vi "Autonomous Independent.vi"() -> ()   [LabVIEW 2013]
doc: "This VI is called when autonomous begins, and will automatically be terminated when autonomous ends. You can carry out timed or sensor driven robot movement independently without needing to return to the caller."
uses:
  Autonomous State.ctl
  <vilib>/Rock Robotics/WPI/Solenoid/WPI_SolenoidValue.ctl
  <vilib>/Rock Robotics/WPI/DriverStation/WPI_DriverStationRobotMode2.ctl
  Robot Global Data.vi
  <vilib>/Rock Robotics/WPI/Solenoid/WPI_SolenoidSetEnum.vi
  <vilib>/Rock Robotics/WPI/RobotDrive/WPI_RobotDriveGetSetRefNum.vi
  <vilib>/Rock Robotics/WPI/RobotDrive/WPI_RobotDriveArcadeDrive_Standard(NoSaturation).vi
panel:
  out "Enum":T1
  # "Be sure to right-click and choose Data Operations>>Make Current Value default if you want to save the array values with the VI"
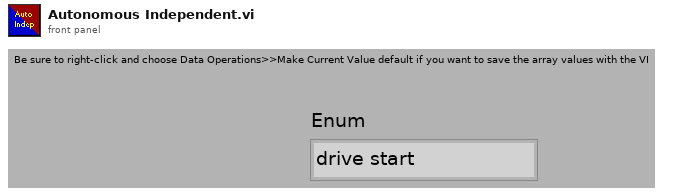
[diagram p1: front panel]
types:
  T1 = typedef "Autonomous State.ctl" = enum16{"drive start", "drive stop", "One Ball: Shoot", "reload", "One Ball: Look for target", "retract arm", "drive faster", "drive time for 2ball", "turn", "One Ball: Finish", "Two Ball: First shoot", "Two Ball: Grab second ball", "Two Ball: Second shoot", "Two Ball: Finish"}
  T2 = typedef "WPI_SolenoidDevRef.ctl" = cluster{"DevStatus":errorcluster, "Solenoid Module":T3, "Forward Solenoid Channel":T4, "Reverse Solenoid Channel":T4}
  T3 = typedef "FPGA_TypedefSolenoidModule.ctl" = enum16{"Solenoid Module 1", "Solenoid Module 2"}
  T4 = typedef "WPI_SolenoidChannel.ctl" = enum8{"Solenoid 1", "Solenoid 2", "Solenoid 3", "Solenoid 4", "Solenoid 5", "Solenoid 6", "Solenoid 7", "Solenoid 8", "Invalid"}
  T5 = typedef "WPI_DriverStationRobotMode2.ctl" = enum16{"Autonomous Disabled", "Autonomous Enabled", "Teleop Disabled", "Teleop Enabled", "Timeout", "Finish", "Test Disabled", "Test Enabled"}
  T6 = typedef "WPI_SolenoidValue.ctl" = enum16{"Off", "On", "Forward", "Reverse"}
  T7 = typedef "WPI_MotorControlDeviceRef.ctl" = cluster{"DeviceStatus":errorcluster, "Type":enum16{"PWM", "CAN"}, "PWM":cluster{"Digital Module":T8, "PWM Channel":T9, "DeadBand":T10}, "CAN":cluster{"Device Number":u8, "Control Mode":T11, "Semaphore":T12, "Max Vout":dbl}, "Invert":bool, "TransformRef":T13, "InvTransformRef":T13}
  T8 = typedef "FPGA_TypedefDigitalModule.ctl" = enum16{"Digital Module 1", "Digital Module 2"}
  T9 = typedef "FPGA_DIOPWMChannel.ctl" = enum8{"PWM 1", "PWM 2", "PWM 3", "PWM 4", "PWM 5", "PWM 6", "PWM 7", "PWM 8", "PWM 9", "PWM 10", "Invalid"}
  T10 = typedef "WPI_PWMDeadband.ctl" = cluster{"Name":string, "maxPositivePwm":i32, "minPositivePwm":i32, "centerPwm":i32, "maxNegativePwm":i32, "minNegativePwm":i32, "angularRange":u16}
  T11 = typedef "WPI_CANJaguar_ControlMode.ctl" = enum8{"Percent VBus", "Current", "Speed", "Position", "Voltage"}
  T12 = typedef "Semaphore RefNum" = refnum<k1>
  T13 = typedef "WPI_PWMTransform_ConPane.ctl" = refnum<vi>
  T14 = typedef "WPI_DigitalInputDevRef.ctl" = cluster{"DevStatus":errorcluster, "DIO Channel":T15, "Digital Module":T8}
  T15 = typedef "FPGA_DIOChannel.ctl" = enum8{"DIO 1", "DIO 2", "DIO 3", "DIO 4", "DIO 5", "DIO 6", "DIO 7", "DIO 8", "DIO 9", "DIO 10", "DIO 11", "DIO 12", "DIO 13", "DIO 14", "Invalid"}
  T16 = typedef "WPI_RobotDriveDevRef.ctl" = cluster{"DevStatus":errorcluster, "Motors[]":T7[], "Square Inputs":bool, "Max Output":dbl, "Isochronous":bool}
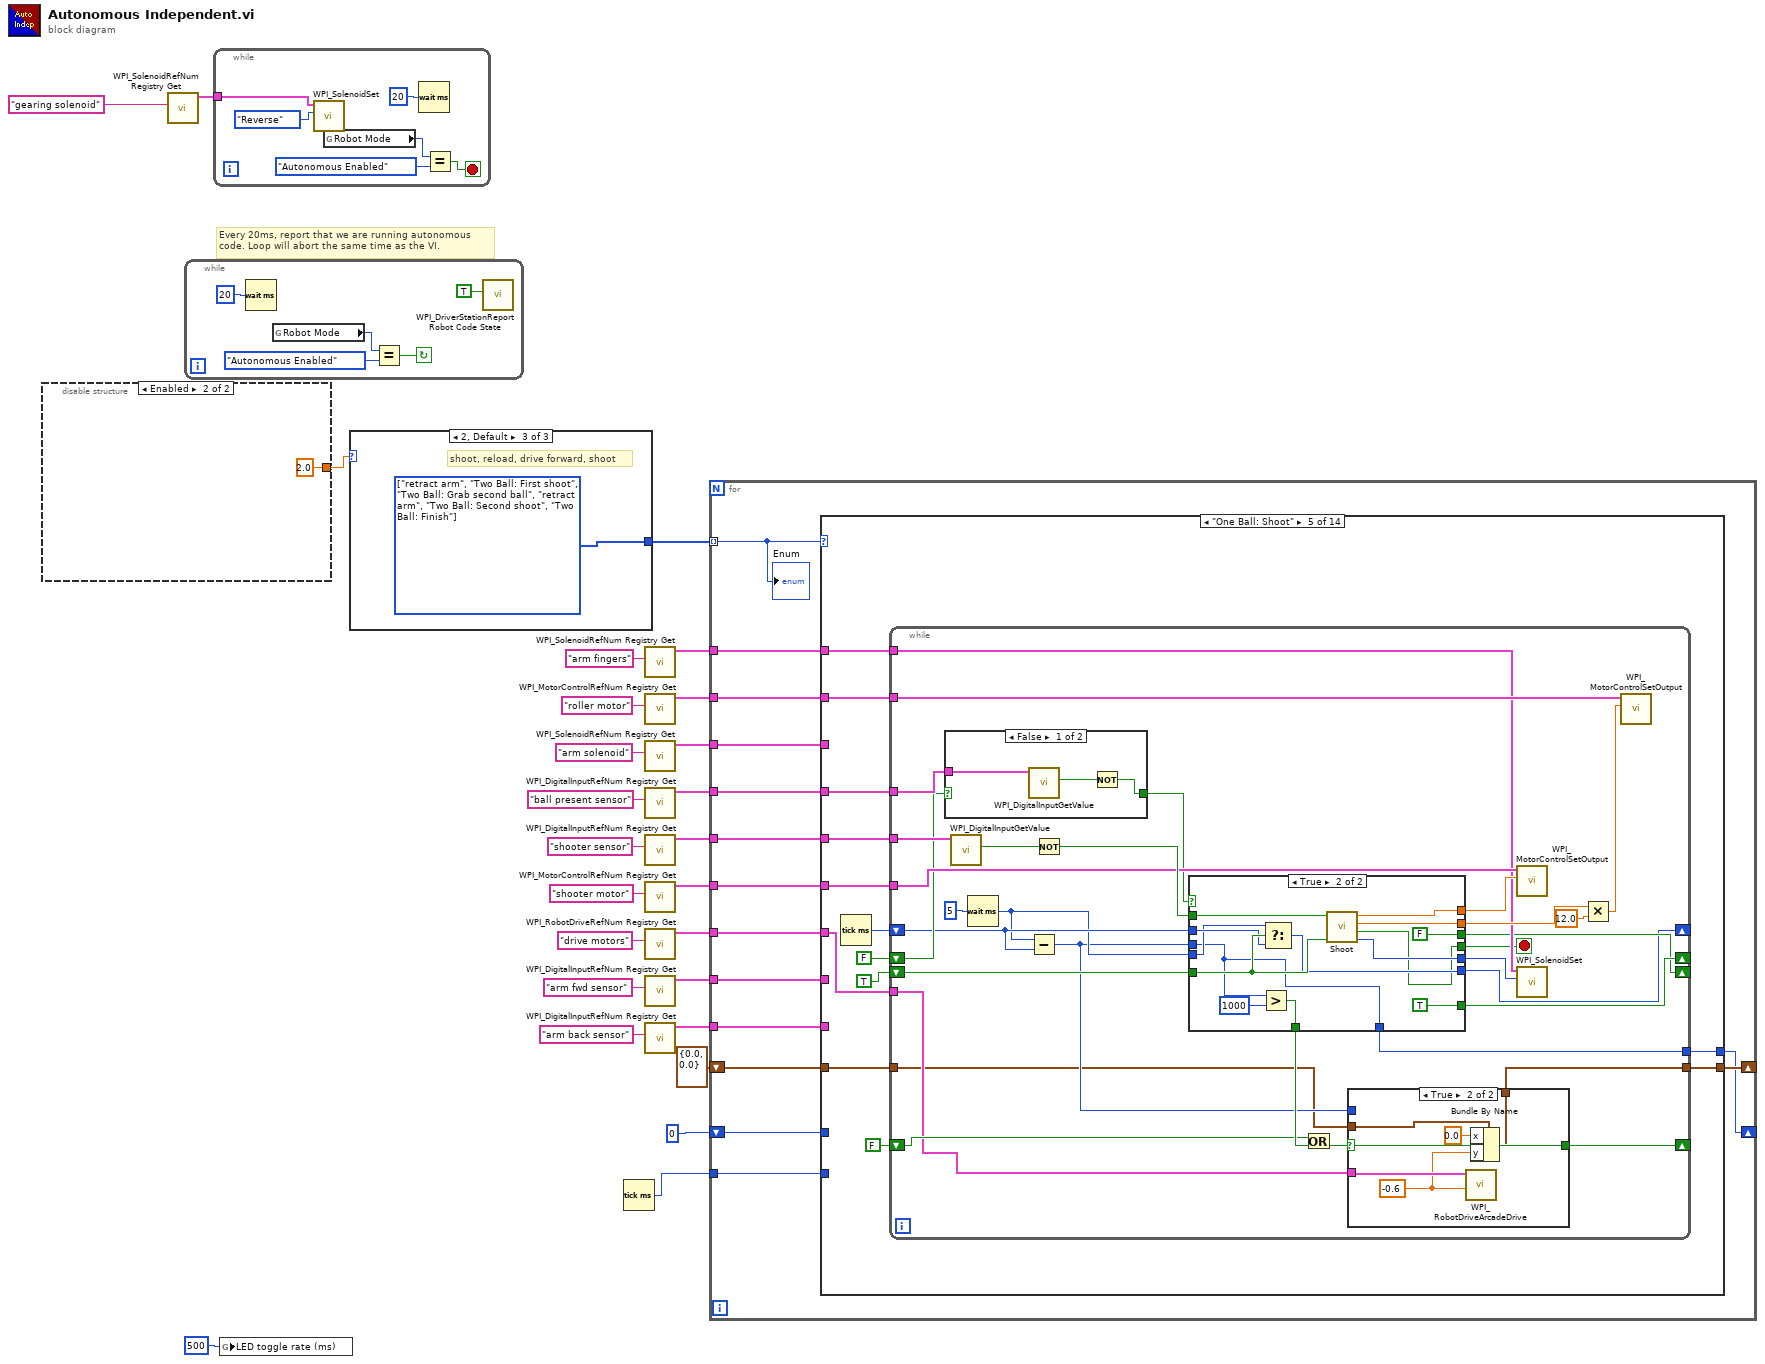
[diagram p0: block diagram]
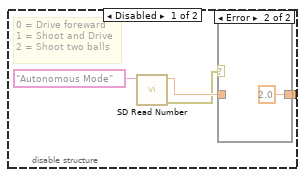
[diagram p2: hidden frame]
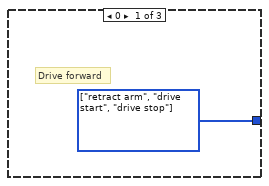
[diagram p4: hidden frame]
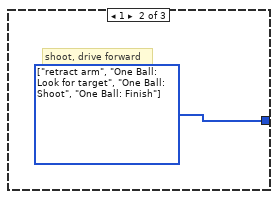
[diagram p5: hidden frame]
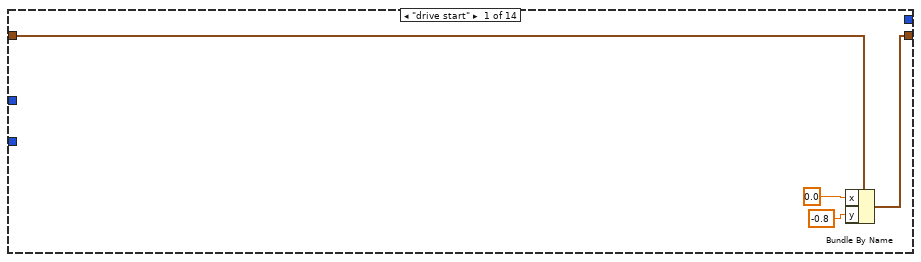
[diagram p6: hidden frame]
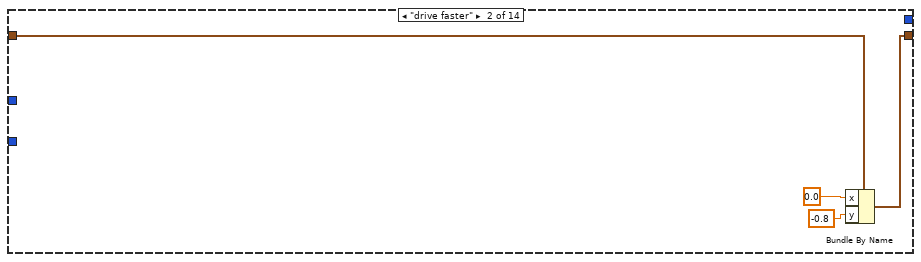
[diagram p7: hidden frame]
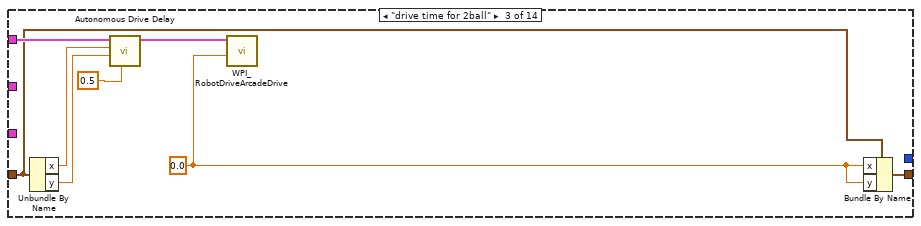
[diagram p8: hidden frame]
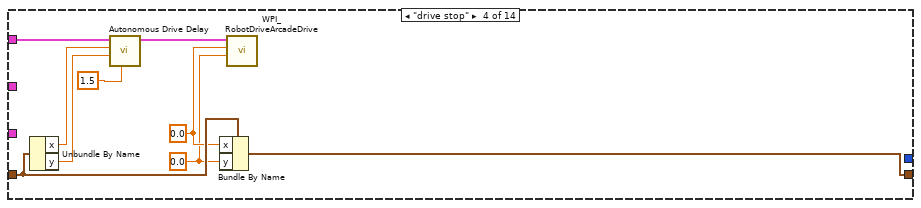
[diagram p9: hidden frame]
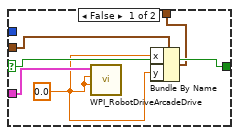
[diagram p10: hidden frame]
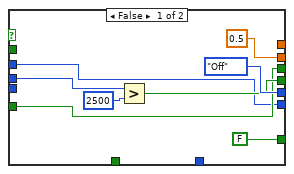
[diagram p12: hidden frame]
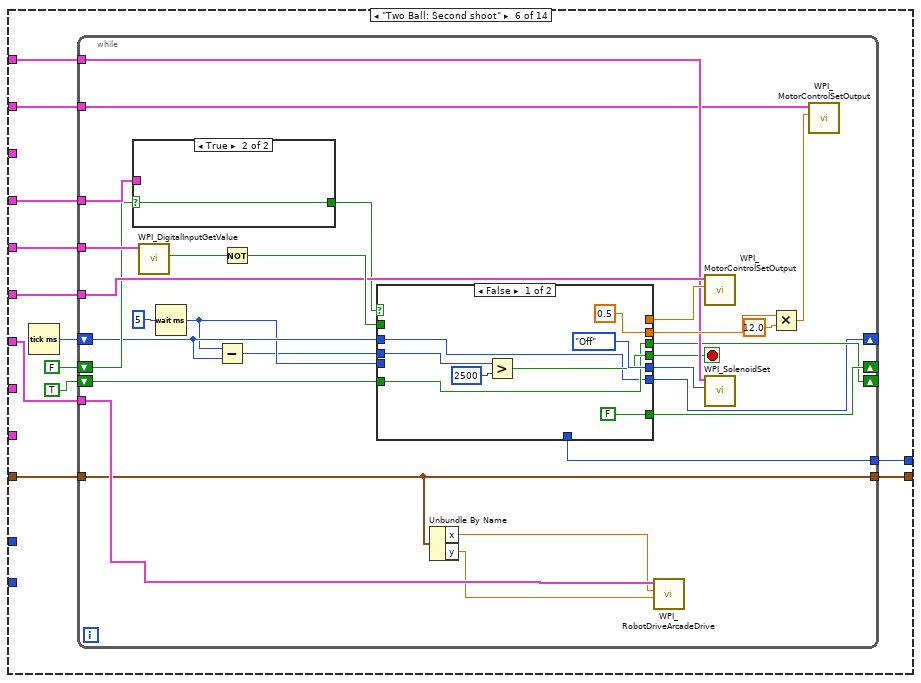
[diagram p13: hidden frame]
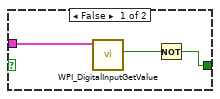
[diagram p14: hidden frame]
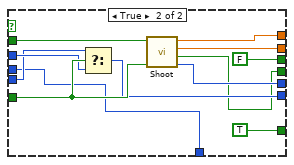
[diagram p15: hidden frame]
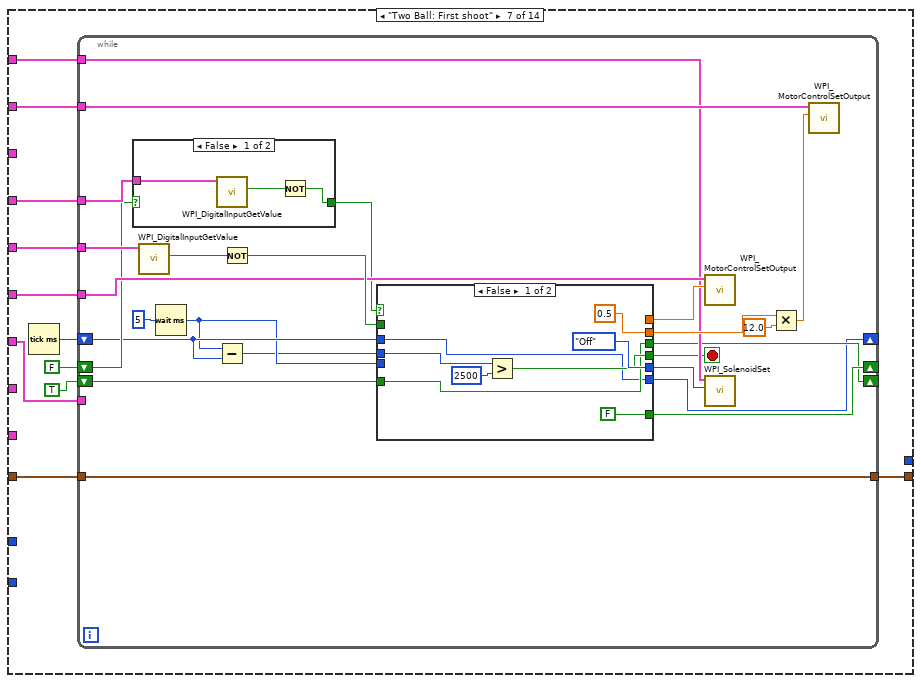
[diagram p16: hidden frame]
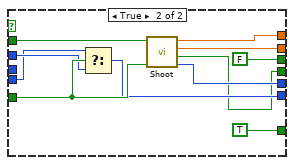
[diagram p18: hidden frame]
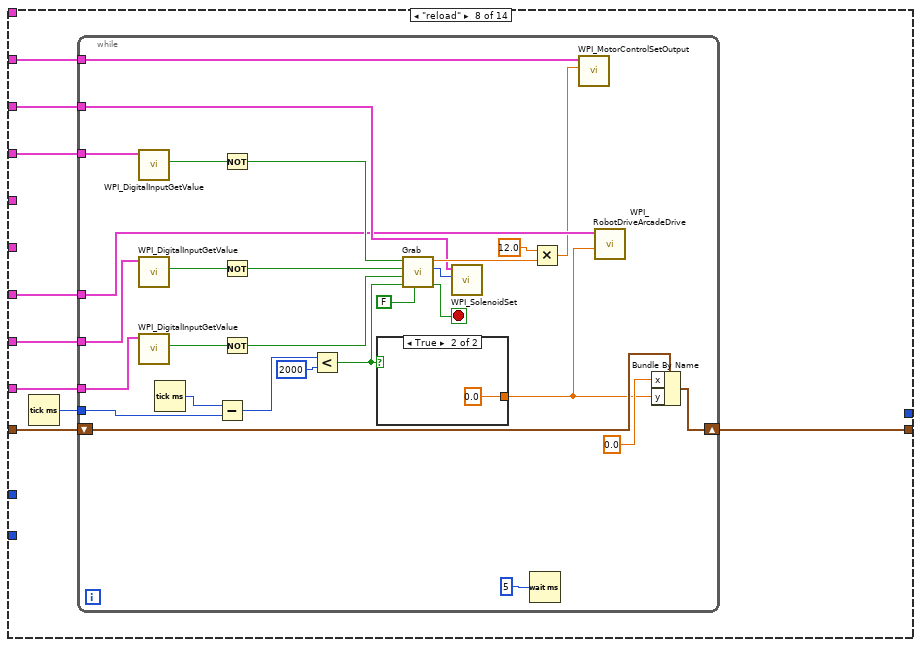
[diagram p19: hidden frame]
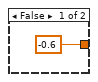
[diagram p20: hidden frame]
diagram:
  # "Every 20ms, report that we are running autonomous\ncode. Loop will abort the same time as the VI."
  n1 = disable-structure shown="Enabled" {
    disable-tunnel: [w29 2.0 ("Numeric")] -> w1
    frame Disabled {
      # "0 = Drive foreward\n1 = Shoot and Drive\n2 = Shoot two balls"
      n2 = call <vilib>:"SD Read Number.vi"("Name"="Autonomous Mode") -> ("error out"=w27:errorcluster, "Numeric"=w28:dbl)  [unwired: 8 in, 1 out]
      n3 = case shown="Error" w27 {
        tunnel: [w31 2.0 ("Numeric")] -> w29
        tunnel: w28 -> [w31 _]
        frame No Error {
        }
        frame Error {
        }
      }
    }
    frame Enabled {
    }
  }
  n4 = call <vilib>:"WPI_SolenoidRefNum Registry Get.vi"("refnum name"="gearing solenoid") -> ("SolenoidDevRef"=w2:T2)  [unwired: 9 in, 1 out]
  n5 = while {
    stop <- w34 continue-if-true
    n6 = Wait (ms)(milliseconds to wait=u32 20) -> ()  [unwired: 1 out]
    n7 = global read "Robot Global Data.vi" "Robot Mode"() -> (w36:T5)
    n8 = Equal?(x=w36, y=WPI_DriverStationRobotMode2."Autonomous Enabled") -> (x = y?=w34:bool)
    n9 = call <vilib>:"WPI_DriverStationReport Robot Code State.vi"("Autonomous"=TRUE) -> ()  [unwired: 10 in, 1 out]
  }
  n10 = while {
    tunnel: w2 -> [w43]
    stop <- w40 stop-if-true
    n11 = call-poly <vilib>:"WPI_SolenoidSet.vi"("Value"=WPI_SolenoidValue."Reverse", "SolenoidDevRef"=w43) -> ()  [unwired: 8 in, 2 out]
    n12 = global read "Robot Global Data.vi" "Robot Mode"() -> (w41:T5)
    n13 = Wait (ms)(milliseconds to wait=u32 20) -> ()  [unwired: 1 out]
    n14 = Equal?(x=w41, y=WPI_DriverStationRobotMode2."Autonomous Enabled") -> (x = y?=w40:bool)
  }
  n15 = global write "Robot Global Data.vi" "LED toggle rate (ms)"(u32 500 ("LED ms toggle rate")) -> ()
  n16 = case shown="2, Default" w1 {
    tunnel: [w45 w46 w47] -> w7
    frame 0 {
      w45 = T1[] [enum."retract arm", enum."drive start", enum."drive stop"] items=["drive start", "drive stop", "One Ball: Shoot", "reload", "One Ball: Look for target", "retract arm", "drive faster", "drive time for 2ball", "turn", "One Ball: Finish", "Two Ball: First shoot", "Two Ball: Grab second ball", "Two Ball: Second shoot", "Two Ball: Finish"]
      # "Drive forward"
    }
    frame 1 {
      w46 = T1[] [enum."retract arm", enum."One Ball: Look for target", enum."One Ball: Shoot", enum."One Ball: Finish"] items=["drive start", "drive stop", "One Ball: Shoot", "reload", "One Ball: Look for target", "retract arm", "drive faster", "drive time for 2ball", "turn", "One Ball: Finish", "Two Ball: First shoot", "Two Ball: Grab second ball", "Two Ball: Second shoot", "Two Ball: Finish"]
      # "shoot, drive forward"
    }
    frame 2, Default {
      w47 = T1[] [enum."retract arm", enum."Two Ball: First shoot", enum."Two Ball: Grab second ball", enum."retract arm", enum."Two Ball: Second shoot", enum."Two Ball: Finish"] items=["drive start", "drive stop", "One Ball: Shoot", "reload", "One Ball: Look for target", "retract arm", "drive faster", "drive time for 2ball", "turn", "One Ball: Finish", "Two Ball: First shoot", "Two Ball: Grab second ball", "Two Ball: Second shoot", "Two Ball: Finish"]
      # "shoot, reload, drive forward, shoot"
    }
  }
  n17 = Tick Count (ms)() -> (millisecond timer value=w4:u32)
  n18 = call <vilib>:"WPI_SolenoidRefNum Registry Get.vi"("refnum name"="arm fingers") -> ("SolenoidDevRef"=w9:T2)  [unwired: 9 in, 1 out]
  n19 = call <vilib>:"WPI_MotorControlRefNum Registry Get.vi"("refnum name"="roller motor") -> ("MotorControlDevRef"=w14:T7)  [unwired: 9 in, 1 out]
  n20 = call <vilib>:"WPI_SolenoidRefNum Registry Get.vi"("refnum name"="arm solenoid") -> ("SolenoidDevRef"=w13:T2)  [unwired: 9 in, 1 out]
  n21 = call <vilib>:"WPI_DigitalInputRefNum Registry Get.vi"("refnum name"="ball present sensor") -> ("DigitalInputDevRef"=w10:T14)  [unwired: 9 in, 1 out]
  n22 = call <vilib>:"WPI_DigitalInputRefNum Registry Get.vi"("refnum name"="shooter sensor") -> ("DigitalInputDevRef"=w16:T14)  [unwired: 9 in, 1 out]
  n23 = call <vilib>:"WPI_MotorControlRefNum Registry Get.vi"("refnum name"="shooter motor") -> ("MotorControlDevRef"=w15:T7)  [unwired: 9 in, 1 out]
  n24 = call <vilib>:"WPI_RobotDriveRefNum Registry Get.vi"("refnum name"="drive motors") -> ("RobotDriveDevRef"=w17:T16)  [unwired: 9 in, 1 out]
  n25 = call <vilib>:"WPI_DigitalInputRefNum Registry Get.vi"("refnum name"="arm fwd sensor") -> ("DigitalInputDevRef"=w11:T14)  [unwired: 9 in, 1 out]
  n26 = call <vilib>:"WPI_DigitalInputRefNum Registry Get.vi"("refnum name"="arm back sensor") -> ("DigitalInputDevRef"=w12:T14)  [unwired: 9 in, 1 out]
  n27 = for {
    tunnel: w7 -> [w62] mode=indexing
    tunnel: w17 -> [w54]
    tunnel: w16 -> [w61]
    tunnel: w15 -> [w60]
    tunnel: w14 -> [w59]
    tunnel: w13 -> [w58]
    tunnel: w12 -> [w57]
    tunnel: w11 -> [w56]
    tunnel: w10 -> [w55]
    tunnel: w9 -> [w53]
    shift-right: [w51] -> _
    shift-left: cluster{"x":dbl, "y":dbl} {"x"=0.0, "y"=0.0} -> [w52]
    shift-right: [w50] -> _
    shift-left: u32 0 -> [w49]
    tunnel: w4 -> [w48]
    n28 = case shown="\"One Ball: Shoot\"" w62 {
      tunnel: w61 -> [_ _ _ _ w100 w180 w243 _ _ _ _ _ _ _]
      tunnel: w60 -> [_ _ _ _ w99 w179 w242 _ _ _ _ _ _ _]
      tunnel: w59 -> [_ _ _ _ w98 w178 w241 w295 w335 _ _ _ _ _]
      tunnel: w58 -> [_ _ _ _ _ _ _ w294 w334 _ w387 _ _ _]
      tunnel: w57 -> [_ _ _ _ _ _ _ w298 w338 _ w386 _ _ _]
      tunnel: w56 -> [_ _ _ _ _ _ _ w297 w337 _ _ _ _ _]
      tunnel: w55 -> [_ _ _ _ w95 w175 w238 w296 w336 _ _ _ _ _]
      tunnel: w54 -> [_ _ w76 w84 w96 w176 w239 w293 w333 _ w385 _ w415 w433]
      tunnel: w53 -> [_ _ _ _ w97 w177 w240 _ _ _ _ _ _ _]
      tunnel: w52 -> [w66 w70 w75 w82 w93 w173 w236 w292 w332 w371 w384 w410 w416 w429]
      tunnel: [w65 w69 w78 w81 w92 w172 w235 w291 w331 w371 w384 w410 w414 w432] -> w51
      tunnel: [_ _ _ _ w88 w169 _ _ _ _ _ _ _ _] -> w50
      tunnel: w49 -> [_ _ _ _ _ _ _ _ _ _ _ _ w411 _]
      tunnel: w48 -> [_ _ _ _ _ _ _ _ _ _ _ _ _ w430]
      frame "drive start" {
        n29 = Bundle By Name(cluster=w66, "x"=0.0 ("X axis value"), "y"=-0.8 ("Y axis value")) -> (w65:cluster{"x":dbl, "y":dbl})
      }
      frame "drive faster" {
        n30 = Bundle By Name(cluster=w70, "x"=0.0, "y"=-0.8 ("Y axis value")) -> (w69:cluster{"x":dbl, "y":dbl})
      }
      frame "drive time for 2ball" {
        w77 = 0.0 ("Y axis value")
        n31 = Unbundle By Name(w75) -> ("x"=w74:dbl, "y"=w73:dbl)
        n32 = call "Autonomous Drive Delay.vi"("Time"=0.5 ("Delay (s)"), "Y"=w73, "X"=w74, "RobotDriveDevRef in"=w76) -> ("RobotDriveDevRef out"=w71:T16)  [unwired: 6 in, 1 out]
        n33 = call-poly <vilib>:"WPI_RobotDriveArcadeDrive.vi"("Y axis value"=w77, "RobotDriveDevRef"=w71) -> ()  [unwired: 7 in, 3 out]
        n34 = Bundle By Name(cluster=w75, "x"=w77, "y"=w77) -> (w78:cluster{"x":dbl, "y":dbl})
      }
      frame "drive stop" {
        w80 = 0.0 ("X axis value")
        w79 = 0.0 ("Y axis value")
        n35 = Unbundle By Name(w82) -> ("x"=w87:dbl, "y"=w86:dbl)
        n36 = call "Autonomous Drive Delay.vi"("Time"=1.5, "Y"=w86, "X"=w87, "RobotDriveDevRef in"=w84) -> ("RobotDriveDevRef out"=w83:T16)  [unwired: 6 in, 1 out]
        n37 = Bundle By Name(cluster=w82, "x"=w80, "y"=w79) -> (w81:cluster{"x":dbl, "y":dbl})
        n38 = call-poly <vilib>:"WPI_RobotDriveArcadeDrive.vi"("Y axis value"=w79, "X axis value"=w80, "RobotDriveDevRef"=w83) -> ()  [unwired: 6 in, 3 out]
      }
      frame "One Ball: Shoot" {
        n39 = Tick Count (ms)() -> (millisecond timer value=w91:u32)
        n40 = while {
          tunnel: w100 -> [w130]
          tunnel: w99 -> [w127]
          tunnel: w98 -> [w125]
          tunnel: w97 -> [w121]
          tunnel: w96 -> [w105]
          tunnel: w95 -> [w118]
          shift-right: [w115] -> _
          shift-left: FALSE -> [w116]
          tunnel: w93 -> [w102]
          tunnel: [w101] -> w92
          shift-right: [w113] -> _
          shift-left: TRUE -> [w114]
          shift-right: [w112] -> _
          shift-left: w91 -> [w111]
          shift-right: [w107] -> _
          shift-left: FALSE -> [w106]
          tunnel: [w104] -> w88
          stop <- w119 stop-if-true
          n41 = case shown="False" w116 {
            selector: w116 -> [_ w146]
            tunnel: w118 -> [w144 _]
            tunnel: [w143 w146] -> w117
            frame False {
              n42 = call <vilib>:"WPI_DigitalInputGetValue.vi"("DigitalInputDevRef"=w144) -> ("Value"=w145:bool)  [unwired: 8 in, 2 out]
              n43 = Not(x=w145) -> (.not. x?=w143:bool)
            }
            frame True {
            }
          }
          n44 = call <vilib>:"WPI_DigitalInputGetValue.vi"("DigitalInputDevRef"=w130) -> ("Value"=w131:bool)  [unwired: 8 in, 2 out]
          n45 = Wait (ms)(milliseconds to wait=u32 5) -> (millisecond timer value=w110:u32)
          n46 = Subtract(x=w110, y=w111) -> (x-y=w103:u32)
          n47 = Not(x=w131) -> (.not. x?=w129:bool)
          n48 = case shown="True" w117 {
            tunnel: w129 -> [_ w168]
            tunnel: [_ w167] -> w126
            tunnel: [0.5 ("Roller Motor Value") w166] -> w124
            tunnel: [WPI_SolenoidValue."Off" ("Arm fingers state") w165] -> w120
            tunnel: [w152 w158] -> w119
            tunnel: [FALSE TRUE] -> w115
            tunnel: w103 -> [w149 w156]
            tunnel: w114 -> [w148 w162]
            tunnel: [w148 FALSE] -> w113
            tunnel: [w147 w161] -> w112
            tunnel: w111 -> [w147 w160]
            tunnel: w110 -> [_ w159]
            tunnel: [_ w157] -> w109
            tunnel: [_ w156] -> w104
            frame False {
              n49 = Greater?(x=w149, y=u32 2500) -> (0:w152:bool)
            }
            frame True {
              n50 = Greater?(x=w156, y=u32 1000) -> (0:w157:bool)
              n51 = Select(t=w159, s=w162, f=w160) -> (s? t:f=w161:u32)
              n52 = call "Shoot.vi"("Reset"=w162, "Shooter Sensor"=w168) -> ("Arm fingers state"=w165:T6, "Finished?"=w158:bool, "Roller Motor Value"=w166:dbl, "Shooter Motor Value"=w167:dbl)  [unwired: 6 in]
            }
          }
          n53 = Or(x=w106, y=w109) -> (x .or. y?=w108:bool)
          n54 = case shown="True" w108 {
            selector: w108 -> [w135 w142]
            tunnel: [w135 w142] -> w107
            tunnel: w105 -> [w136 w141]
            tunnel: w103 -> [_ _]
            tunnel: w102 -> [w134 w140]
            tunnel: [w133 w139] -> w101
            frame False {
              w132 = 0.0 ("Delay (s)")
              n55 = call-poly <vilib>:"WPI_RobotDriveArcadeDrive.vi"("Y axis value"=w132, "X axis value"=w132, "RobotDriveDevRef"=w136) -> ()  [unwired: 6 in, 3 out]
              n56 = Bundle By Name(cluster=w134, "x"=w132, "y"=w132) -> (w133:cluster{"x":dbl, "y":dbl})
            }
            frame True {
              w138 = -0.6 ("Y axis value")
              n57 = call-poly <vilib>:"WPI_RobotDriveArcadeDrive.vi"("Y axis value"=w138, "RobotDriveDevRef"=w141) -> ()  [unwired: 7 in, 3 out]
              n58 = Bundle By Name(cluster=w140, "x"=0.0, "y"=w138) -> (w139:cluster{"x":dbl, "y":dbl})
            }
          }
          n59 = call <vilib>:"WPI_MotorControlSetOutput.vi"("Output"=w126, "MotorControlDevRef"=w127) -> ()  [unwired: 7 in, 3 out]
          n60 = call-poly <vilib>:"WPI_SolenoidSet.vi"("Value"=w120, "SolenoidDevRef"=w121) -> ()  [unwired: 8 in, 2 out]
          n61 = Multiply(x=w124, y=12.0) -> (x*y=w123:dbl)
          n62 = call <vilib>:"WPI_MotorControlSetOutput.vi"("Output"=w123, "MotorControlDevRef"=w125) -> ()  [unwired: 7 in, 3 out]
        }
      }
      frame "Two Ball: Second shoot" {
        n63 = Tick Count (ms)() -> (millisecond timer value=w171:u32)
        n64 = while {
          tunnel: w180 -> [w207]
          tunnel: w179 -> [w204]
          tunnel: w178 -> [w181]
          tunnel: w177 -> [w199]
          tunnel: w176 -> [w187]
          tunnel: w175 -> [w196]
          shift-right: [w193] -> _
          shift-left: FALSE -> [w194]
          tunnel: w173 -> [w184]
          tunnel: [w184] -> w172
          shift-right: [w191] -> _
          shift-left: TRUE -> [w192]
          shift-right: [w190] -> _
          shift-left: w171 -> [w189]
          tunnel: [w186] -> w169
          stop <- w197 stop-if-true
          n65 = case shown="True" w194 {
            selector: w194 -> [_ w212]
            tunnel: w196 -> [w210 _]
            tunnel: [w209 w212] -> w195
            frame False {
              n66 = call <vilib>:"WPI_DigitalInputGetValue.vi"("DigitalInputDevRef"=w210) -> ("Value"=w211:bool)  [unwired: 8 in, 2 out]
              n67 = Not(x=w211) -> (.not. x?=w209:bool)
            }
            frame True {
            }
          }
          n68 = call <vilib>:"WPI_DigitalInputGetValue.vi"("DigitalInputDevRef"=w207) -> ("Value"=w208:bool)  [unwired: 8 in, 2 out]
          n69 = Wait (ms)(milliseconds to wait=u32 5) -> (millisecond timer value=w188:u32)
          n70 = Subtract(x=w188, y=w189) -> (x-y=w185:u32)
          n71 = Not(x=w208) -> (.not. x?=w206:bool)
          n72 = case shown="False" w195 {
            tunnel: w206 -> [_ w232]
            tunnel: [_ w231] -> w203
            tunnel: [0.5 ("Roller Motor Value") w230] -> w202
            tunnel: [WPI_SolenoidValue."Off" ("Arm fingers state") w229] -> w198
            tunnel: [w218 w222] -> w197
            tunnel: [FALSE TRUE] -> w193
            tunnel: w185 -> [w215 w221]
            tunnel: w192 -> [w214 w226]
            tunnel: [w214 FALSE] -> w191
            tunnel: [w213 w225] -> w190
            tunnel: w189 -> [w213 w224]
            tunnel: w188 -> [_ w223]
            tunnel: [_ w221] -> w186
            frame False {
              n73 = Greater?(x=w215, y=u32 2500) -> (0:w218:bool)
            }
            frame True {
              n74 = Select(t=w223, s=w226, f=w224) -> (s? t:f=w225:u32)
              n75 = call "Shoot.vi"("Reset"=w226, "Shooter Sensor"=w232) -> ("Arm fingers state"=w229:T6, "Finished?"=w222:bool, "Roller Motor Value"=w230:dbl, "Shooter Motor Value"=w231:dbl)  [unwired: 6 in]
            }
          }
          n76 = Unbundle By Name(w184) -> ("x"=w183:dbl, "y"=w182:dbl)
          n77 = call-poly <vilib>:"WPI_RobotDriveArcadeDrive.vi"("Y axis value"=w182, "X axis value"=w183, "RobotDriveDevRef"=w187) -> ()  [unwired: 6 in, 3 out]
          n78 = call <vilib>:"WPI_MotorControlSetOutput.vi"("Output"=w203, "MotorControlDevRef"=w204) -> ()  [unwired: 7 in, 3 out]
          n79 = call-poly <vilib>:"WPI_SolenoidSet.vi"("Value"=w198, "SolenoidDevRef"=w199) -> ()  [unwired: 8 in, 2 out]
          n80 = Multiply(x=w202, y=12.0) -> (x*y=w201:dbl)
          n81 = call <vilib>:"WPI_MotorControlSetOutput.vi"("Output"=w201, "MotorControlDevRef"=w181) -> ()  [unwired: 7 in, 3 out]
        }
      }
      frame "Two Ball: First shoot" {
        n82 = Tick Count (ms)() -> (millisecond timer value=w234:u32)
        n83 = while {
          tunnel: w243 -> [w266]
          tunnel: w242 -> [w263]
          tunnel: w241 -> [w261]
          tunnel: w240 -> [w257]
          tunnel: w239 -> [_]
          tunnel: w238 -> [w254]
          shift-right: [w251] -> _
          shift-left: FALSE -> [w252]
          tunnel: w236 -> [w250]
          tunnel: [w250] -> w235
          shift-right: [w248] -> _
          shift-left: TRUE -> [w249]
          shift-right: [w247] -> _
          shift-left: w234 -> [w246]
          stop <- w255 stop-if-true
          n84 = case shown="False" w252 {
            selector: w252 -> [_ w271]
            tunnel: w254 -> [w269 _]
            tunnel: [w268 w271] -> w253
            frame False {
              n85 = call <vilib>:"WPI_DigitalInputGetValue.vi"("DigitalInputDevRef"=w269) -> ("Value"=w270:bool)  [unwired: 8 in, 2 out]
              n86 = Not(x=w270) -> (.not. x?=w268:bool)
            }
            frame True {
            }
          }
          n87 = call <vilib>:"WPI_DigitalInputGetValue.vi"("DigitalInputDevRef"=w266) -> ("Value"=w267:bool)  [unwired: 8 in, 2 out]
          n88 = Wait (ms)(milliseconds to wait=u32 5) -> (millisecond timer value=w245:u32)
          n89 = Subtract(x=w245, y=w246) -> (x-y=w244:u32)
          n90 = Not(x=w267) -> (.not. x?=w265:bool)
          n91 = case shown="False" w253 {
            tunnel: w265 -> [_ w290]
            tunnel: [_ w289] -> w262
            tunnel: [0.5 ("Roller Motor Value") w288] -> w260
            tunnel: [WPI_SolenoidValue."Off" ("Arm fingers state") w287] -> w256
            tunnel: [w277 w280] -> w255
            tunnel: [FALSE TRUE] -> w251
            tunnel: w244 -> [w274 _]
            tunnel: w249 -> [w273 w284]
            tunnel: [w273 FALSE] -> w248
            tunnel: [w272 w283] -> w247
            tunnel: w246 -> [w272 w282]
            tunnel: w245 -> [_ w281]
            frame False {
              n92 = Greater?(x=w274, y=u32 2500) -> (0:w277:bool)
            }
            frame True {
              n93 = Select(t=w281, s=w284, f=w282) -> (s? t:f=w283:u32)
              n94 = call "Shoot.vi"("Reset"=w284, "Shooter Sensor"=w290) -> ("Arm fingers state"=w287:T6, "Finished?"=w280:bool, "Roller Motor Value"=w288:dbl, "Shooter Motor Value"=w289:dbl)  [unwired: 6 in]
            }
          }
          n95 = call <vilib>:"WPI_MotorControlSetOutput.vi"("Output"=w262, "MotorControlDevRef"=w263) -> ()  [unwired: 7 in, 3 out]
          n96 = call-poly <vilib>:"WPI_SolenoidSet.vi"("Value"=w256, "SolenoidDevRef"=w257) -> ()  [unwired: 8 in, 2 out]
          n97 = Multiply(x=w260, y=12.0) -> (x*y=w259:dbl)
          n98 = call <vilib>:"WPI_MotorControlSetOutput.vi"("Output"=w259, "MotorControlDevRef"=w261) -> ()  [unwired: 7 in, 3 out]
        }
      }
      frame "reload" {
        n99 = Tick Count (ms)() -> (millisecond timer value=w299:u32)
        n100 = while {
          tunnel: w299 -> [w325]
          tunnel: w298 -> [w320]
          tunnel: w297 -> [w317]
          tunnel: w296 -> [w314]
          tunnel: w295 -> [w310]
          tunnel: w294 -> [w309]
          tunnel: w293 -> [w306]
          shift-right: [w300] -> w291
          shift-left: w292 -> [w303]
          stop <- w326 stop-if-true
          n101 = call <vilib>:"WPI_DigitalInputGetValue.vi"("DigitalInputDevRef"=w314) -> ("Value"=w315:bool)  [unwired: 8 in, 2 out]
          n102 = call <vilib>:"WPI_DigitalInputGetValue.vi"("DigitalInputDevRef"=w317) -> ("Value"=w318:bool)  [unwired: 8 in, 2 out]
          n103 = call <vilib>:"WPI_DigitalInputGetValue.vi"("DigitalInputDevRef"=w320) -> ("Value"=w321:bool)  [unwired: 8 in, 2 out]
          n104 = Tick Count (ms)() -> (millisecond timer value=w324:u32)
          n105 = Subtract(x=w324, y=w325) -> (x-y=w323:u32)
          n106 = Not(x=w315) -> (.not. x?=w313:bool)
          n107 = Not(x=w318) -> (.not. x?=w316:bool)
          n108 = Not(x=w321) -> (.not. x?=w319:bool)
          n109 = Less?(x=w323, y=u32 2000) -> (x < y?=w307:bool)
          n110 = case shown="True" w307 {
            tunnel: [-0.6 0.0] -> w301
            frame False {
            }
            frame True {
            }
          }
          n111 = call "Grab.vi"("Reset"=FALSE, "Button Pressed?"=w307, "Arm Back?"=w319, "Arm Forward?"=w316, "Ball Present?"=w313) -> ("Finished?"=w326:bool, "Arm state"=w312:T6, "Roller Speed"=w311:dbl)  [unwired: 4 in]
          n112 = call-poly <vilib>:"WPI_SolenoidSet.vi"("Value"=w312, "SolenoidDevRef"=w309) -> ()  [unwired: 8 in, 2 out]
          n113 = Wait (ms)(milliseconds to wait=u32 5) -> ()  [unwired: 1 out]
          n114 = Multiply(x=12.0, y=w311) -> (x*y=w305:dbl)
          n115 = call <vilib>:"WPI_MotorControlSetOutput.vi"("Output"=w305, "MotorControlDevRef"=w310) -> ()  [unwired: 7 in, 3 out]
          n116 = call-poly <vilib>:"WPI_RobotDriveArcadeDrive.vi"("Y axis value"=w301, "RobotDriveDevRef"=w306) -> ()  [unwired: 7 in, 3 out]
          n117 = Bundle By Name(cluster=w303, "x"=0.0, "y"=w301) -> (w300:cluster{"x":dbl, "y":dbl})
        }
      }
      frame "Two Ball: Grab second ball" {
        n118 = Tick Count (ms)() -> (millisecond timer value=w339:u32)
        n119 = while {
          tunnel: w339 -> [w367]
          tunnel: w338 -> [w363]
          tunnel: w337 -> [w360]
          tunnel: w336 -> [w357]
          tunnel: w335 -> [w353]
          tunnel: w334 -> [w352]
          tunnel: w333 -> [w349]
          shift-right: [w343] -> w331
          shift-left: w332 -> [w346]
          shift-right: [FALSE ("Reset")] -> _
          shift-left: TRUE ("Reset") -> [w342]
          stop <- w368 stop-if-true
          n120 = Wait (ms)(milliseconds to wait=u32 5) -> (millisecond timer value=w340:u32)
          n121 = call <vilib>:"WPI_DigitalInputGetValue.vi"("DigitalInputDevRef"=w357) -> ("Value"=w358:bool)  [unwired: 8 in, 2 out]
          n122 = call <vilib>:"WPI_DigitalInputGetValue.vi"("DigitalInputDevRef"=w360) -> ("Value"=w361:bool)  [unwired: 8 in, 2 out]
          n123 = call <vilib>:"WPI_DigitalInputGetValue.vi"("DigitalInputDevRef"=w363) -> ("Value"=w364:bool)  [unwired: 8 in, 2 out]
          n124 = Subtract(x=w340, y=w367) -> (x-y=w366:u32)
          n125 = Not(x=w358) -> (.not. x?=w356:bool)
          n126 = Not(x=w361) -> (.not. x?=w359:bool)
          n127 = Not(x=w364) -> (.not. x?=w362:bool)
          n128 = Less?(x=w366, y=u32 2000) -> (x < y?=w350:bool)
          n129 = case shown="True" w350 {
            tunnel: [-0.6 0.0] -> w344
            frame False {
            }
            frame True {
            }
          }
          n130 = call "Grab.vi"("Reset"=w342, "Button Pressed?"=w350, "Arm Back?"=w362, "Arm Forward?"=w359, "Ball Present?"=w356) -> ("Finished?"=w368:bool, "Arm state"=w355:T6, "Roller Speed"=w354:dbl)  [unwired: 4 in]
          n131 = call-poly <vilib>:"WPI_SolenoidSet.vi"("Value"=w355, "SolenoidDevRef"=w352) -> ()  [unwired: 8 in, 2 out]
          n132 = Multiply(x=12.0, y=w354) -> (x*y=w348:dbl)
          n133 = call <vilib>:"WPI_MotorControlSetOutput.vi"("Output"=w348, "MotorControlDevRef"=w353) -> ()  [unwired: 7 in, 3 out]
          n134 = call-poly <vilib>:"WPI_RobotDriveArcadeDrive.vi"("Y axis value"=w344, "RobotDriveDevRef"=w349) -> ()  [unwired: 7 in, 3 out]
          n135 = Bundle By Name(cluster=w346, "x"=0.0, "y"=w344) -> (w343:cluster{"x":dbl, "y":dbl})
        }
      }
      frame "One Ball: Look for target" {
        n136 = Tick Count (ms)() -> (millisecond timer value=w372:u32)
        n137 = while {
          tunnel: w372 -> [w380]
          stop <- w375 stop-if-true
          n138 = Wait (ms)(milliseconds to wait=u32 5) -> ()  [unwired: 1 out]
          n139 = Tick Count (ms)() -> (millisecond timer value=w373:u32)
          n140 = Subtract(x=w373, y=w380) -> (x-y=w379:u32)
          n141 = Greater?(x=w379, y=u32 4500) -> (0:w376:bool)
          n142 = call <vilib>:"SD Read Boolean.vi"("Name"="Target Found") -> ("Boolean"=w377:bool)  [unwired: 8 in, 2 out]
          n143 = Or(x=w377, y=w376) -> (x .or. y?=w375:bool)
        }
      }
      frame "retract arm", Default {
        n144 = while {
          tunnel: w387 -> [w409]
          tunnel: w386 -> [w406]
          tunnel: w385 -> [w405]
          tunnel: [w404] -> _
          tunnel: w384 -> [w403]
          tunnel: [w399] -> w383
          tunnel: [w398] -> w382
          stop <- w407 continue-if-true
          n145 = Unbundle By Name(w403) -> ("x"=w402:dbl, "y"=w401:dbl)
          n146 = call <vilib>:"WPI_DigitalInputGetValue.vi"("DigitalInputDevRef"=w406) -> ("error out"=w404:errorcluster, "Value"=w407:bool)  [unwired: 8 in, 1 out]
          n147 = call-poly <vilib>:"WPI_RobotDriveArcadeDrive.vi"("Y axis value"=w401, "X axis value"=w402, "RobotDriveDevRef"=w405) -> ("RobotDriveDevRef"=w398:T16)  [unwired: 6 in, 2 out]
          n148 = Wait (ms)(milliseconds to wait=u32 5) -> (millisecond timer value=w399:u32)
          n149 = call-poly <vilib>:"WPI_SolenoidSet.vi"("Value"=WPI_SolenoidValue."Forward", "SolenoidDevRef"=w409) -> ()  [unwired: 8 in, 2 out]
        }
        n150 = while {
          tunnel: w384 -> [w396]
          tunnel: w383 -> [w395]
          tunnel: w382 -> [w390]
          stop <- w388 stop-if-true
          n151 = Unbundle By Name(w396) -> ("x"=w391:dbl, "y"=w392:dbl)
          n152 = Wait (ms)(milliseconds to wait=u32 5) -> (millisecond timer value=w394:u32)
          n153 = call-poly <vilib>:"WPI_RobotDriveArcadeDrive.vi"("Y axis value"=w392, "X axis value"=w391, "RobotDriveDevRef"=w390) -> ()  [unwired: 6 in, 3 out]
          n154 = Subtract(x=w394, y=w395) -> (x-y=w393:u32)
          n155 = Greater?(x=w393, y=u32 250) -> (0:w388:bool)
        }
      }
      frame "turn" {
      }
      frame "One Ball: Finish" {
        w413 = 0.0 ("x")
        n156 = Tick Count (ms)() -> (millisecond timer value=w412:u32)
        n157 = while {
          tunnel: w415 -> [w425]
          tunnel: w412 -> [w423]
          tunnel: w411 -> [w421]
          stop <- w418 stop-if-true
          n158 = Wait (ms)(milliseconds to wait=u32 5) -> (millisecond timer value=w424:u32)
          n159 = call-poly <vilib>:"WPI_RobotDriveArcadeDrive.vi"("RobotDriveDevRef"=w425) -> ()  [unwired: 8 in, 3 out]
          n160 = Subtract(x=w424, y=w423) -> (x-y=w422:u32)
          n161 = Add(x=w422, y=w421) -> (x+y=w420:u32)
          n162 = Greater?(x=w420, y=u32 1500) -> (0:w418:bool)
        }
        n163 = Bundle By Name(cluster=w416, "x"=w413, "y"=w413) -> (w414:cluster{"x":dbl, "y":dbl})
      }
      frame "Two Ball: Finish" {
        w431 = 0.0 ("x")
        n164 = Unbundle By Name(w429) -> ("x"=w428:dbl, "y"=w427:dbl)
        n165 = while {
          tunnel: w433 -> [w442]
          tunnel: w430 -> [w440]
          tunnel: w428 -> [w437]
          tunnel: w427 -> [w436]
          tunnel: [w434] -> w426
          stop <- w438 stop-if-true
          n166 = Tick Count (ms)() -> (millisecond timer value=w441:u32)
          n167 = call-poly <vilib>:"WPI_RobotDriveArcadeDrive.vi"("Y axis value"=w436, "X axis value"=w437, "RobotDriveDevRef"=w442) -> ("RobotDriveDevRef"=w434:T16)  [unwired: 6 in, 2 out]
          n168 = Subtract(x=w441, y=w440) -> (x-y=w439:u32)
          n169 = Greater?(x=w439, y=u32 10000) -> (0:w438:bool)
        }
        n170 = Bundle By Name(cluster=w429, "x"=w431, "y"=w431) -> (w432:cluster{"x":dbl, "y":dbl})
        n171 = call-poly <vilib>:"WPI_RobotDriveArcadeDrive.vi"("RobotDriveDevRef"=w426) -> ()  [unwired: 8 in, 3 out]
      }
    }
    "Enum" <- w62
  }
